vi "ClusterOR.vi"(0 "Mod":T1=enum."Bounce") -> (1 "selection?":bool, 2 "disable":i32)   [LabVIEW 2012]
uses:
  SlideParams.ctl
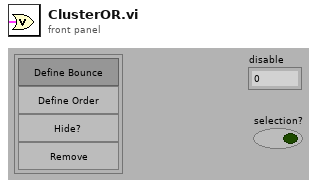
[diagram p1: front panel]
types:
  T1 = typedef "SlideParams.ctl" = enum32{"No Selection", "Bounce", "Order", "Hide", "Remove"}
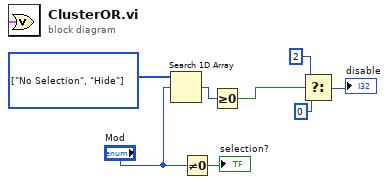
[diagram p0: block diagram]
diagram:
  w4 = T1[] [enum."No Selection", enum."Hide"] items=["No Selection", "Bounce", "Order", "Hide", "Remove"]
  n1 = Search 1D Array(1D array=w4, element="Mod") -> (index of element=w3:i32)  [unwired: 1 in]
  n2 = Not Equal To 0?(x="Mod") -> (x != 0?=→"selection?":bool)
  n3 = Greater Or Equal To 0?(x=w3) -> (x >= 0?=w1:bool)
  n4 = Select(t=2 ("col"), s=w1, f=0 ("col")) -> (s? t:f=→"disable":i32)
